vi "1 Tap 8-Bit.vi"() -> (0 "Pixels":cluster{"Pixel 0":u8})   [LabVIEW 2013]
uses:
  <vilib>/rvi/eio/common/nirviEmuTemplateMethod_errors.vi
  <vilib>/eio/EIONode/EIONode.xnode
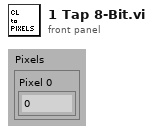
[diagram p1: front panel]
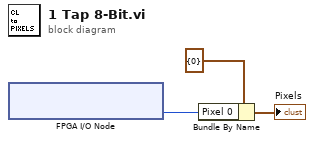
[diagram p0: block diagram]
diagram:
  n1 = xnode "FPGA I/O Node"() -> ("IO Module\\CL Port A"=w2:u8)  [unwired: 1 in, 1 out]
  n2 = Bundle By Name(cluster=cluster{"Pixel 0":u8} {"Pixel 0"=0} ("Data"), "Pixel 0"=w2) -> (→"Pixels":cluster{"Pixel 0":u8})
